vi "Init Array of Motor Config Objs.vi"(8 "error in (no error)":errorcluster, 11 "Motions Configuration in":refnum<class "Motions Configuration.lvclass">) -> (0 "error out":errorcluster, 2 "Array of Motor Config Objs":refnum<class "Motor Configuration.lvclass">[](array[class]), 3 "Motions Configuration out":refnum<class "Motions Configuration.lvclass">)   [LabVIEW 2016, in "Hardware.lvlib" / "Motions.lvlib" / "Motions Configuration.lvclass"]
uses:
  <userlib>/Common Components/Hardware/Abstract System/Motions/Motions Config/Motions Configuration.lvclass
  C:/Program Files (x86)/National Instruments/LabVIEW 2016/user.lib/Configuration Dialog Actor/Configuration.lvclass
  <userlib>/Common Components/Hardware/Motor/Motor Config/Motor Configuration.lvclass
  <userlib>/Common Components/Hardware/Abstract System/Motions/Motions Config/Motions Configuration.lvclass/Motions Configuration.ctl
  <userlib>/Configuration Dialog Actor/Configuration.lvclass/Configuration.ctl
  <userlib>/Common Components/Hardware/Abstract System/Motions/Motions/Motions.lvclass/Motions.ctl
  <userlib>/Common Components/Hardware/Motor/Motor Config/Motor Configuration.lvclass/Motor Configuration.ctl
  <userlib>/Configuration Dialog Actor/Accessors/Write Change Display.vi
  <userlib>/Configuration Dialog Actor/Accessors/Write Sub Panel.vi
  <userlib>/Configuration Dialog Actor/Accessors/Write Title.vi
  <userlib>/Configuration Dialog Actor/Accessors/Write Categories.vi
  <userlib>/Common Components/Hardware/Abstract System/Motions/Motions Config/Read Motions Obj.vi
  <userlib>/Configuration Dialog Actor/Accessors/Read Change Display.vi
  <userlib>/Configuration Dialog Actor/Accessors/Read Sub Panel.vi
  <userlib>/Configuration Dialog Actor/Accessors/Read Title.vi
  <userlib>/Configuration Dialog Actor/Accessors/Read Categories.vi
  <userlib>/Common Components/Hardware/Motor/Motor Config/Accessors/Write Motor Obj.vi
  <userlib>/Common Components/Hardware/Abstract System/Motions/Motions/Motions.lvclass
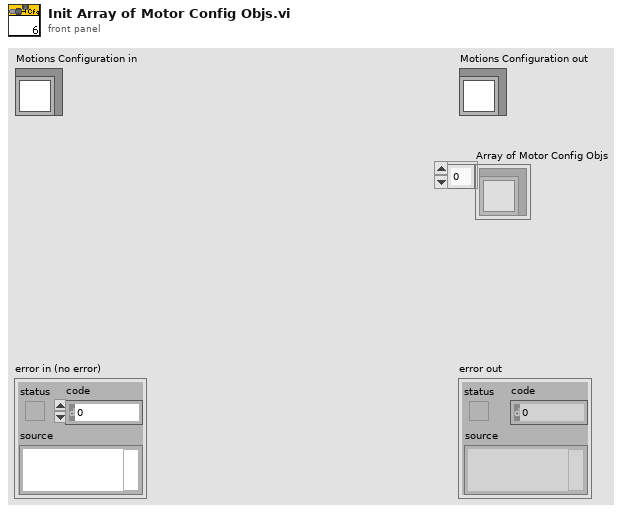
[diagram p1: front panel]
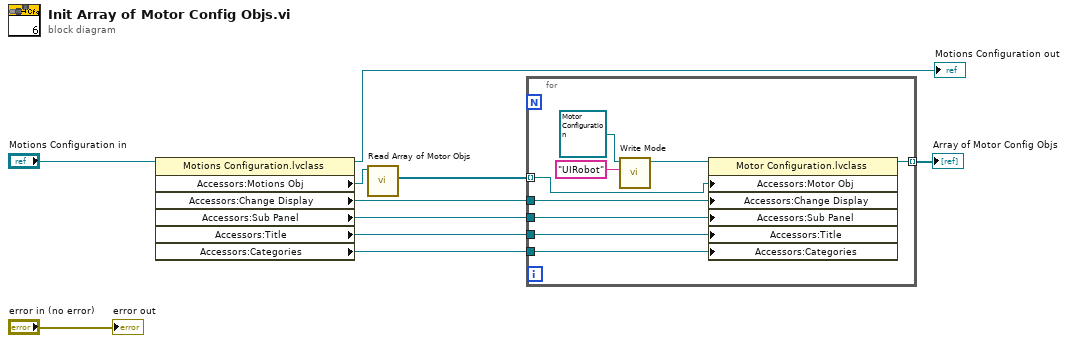
[diagram p0: block diagram]
diagram:
  n1 = property class="Motions Configuration.lvclass"(reference="Motions Configuration in") -> (reference out=→"Motions Configuration out":refnum<class "Motions Configuration.lvclass">, "Accessors:Motions Obj"=w5:refnum<class "Motions.lvclass">, "Accessors:Change Display"=w9:refnum<user-event>, "Accessors:Sub Panel"=w8:refnum<vi>, "Accessors:Title"=w7:refnum<vi>, "Accessors:Categories"=w6:refnum<vi>)  [unwired: 1 in, 1 out]
  n2 = call <userlib>:"Read Array of Motor Objs.vi"("Motions in"=w5) -> ("Array of Motor Objs"=w4:refnum<class "Motor.lvclass">[])  [unwired: 9 in, 1 out]
  n3 = for {
    tunnel: w9 -> [w19]
    tunnel: w8 -> [w18]
    tunnel: w7 -> [w17]
    tunnel: w6 -> [w16]
    tunnel: [w15] -> w1 mode=indexing
    tunnel: w4 -> [w13] mode=indexing
    n4 = call <userlib>:"Write Mode.vi"("Mode"="UIRobot", "Motor Configuration in"=refnum<class "Motor Configuration.lvclass"> refnum ("Hardware.lvlib:Motor.lvlib:Motor Configuration.lvclass")) -> ("Motor Configuration out"=w12:refnum<class "Motor Configuration.lvclass">)  [unwired: 9 in]
    n5 = property class="Motor Configuration.lvclass"(reference=w12, "Accessors:Motor Obj"=w13, "Accessors:Change Display"=w19, "Accessors:Sub Panel"=w18, "Accessors:Title"=w17, "Accessors:Categories"=w16) -> (reference out=w15:refnum<class "Motor Configuration.lvclass">)  [unwired: 1 in, 1 out]
  }
  "Array of Motor Config Objs" <- w1
  "error out" <- "error in (no error)"
